vi "Check Result of the actuation.vi"(8 "error in":errorcluster, 10 "Actuator name":string, 11 "UTP IO Session in":T1) -> (0 "error out":errorcluster, 2 "Result":i16, 3 "UTP IO Session out":T1)   [LabVIEW 2023, in "Actuators.lvlib"]
doc: "Check result of the actuation"
uses:
  Actuators.lvlib
  <vilib>/Noffz/UTP IO/UTP IO Library/Typedefs/Session Handle.ctl
  <vilib>/Noffz/UTP IO/UTP IO Library/UTP IO Pool Session.lvclass
  <vilib>/Noffz/UTP IO/UTP IO Library/methods/poly/plc/Read PLC Variable (I16).vi
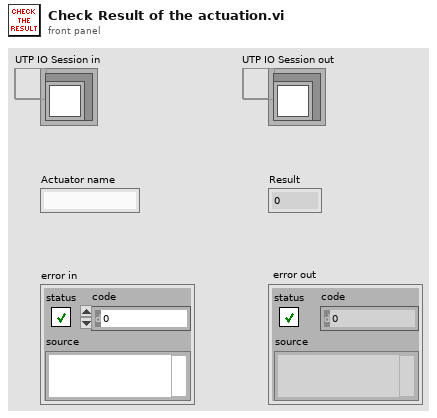
[diagram p1: front panel]
types:
  T1 = typedef "UTP IO Library.lvlib/UTP IO Pool Session.lvclass/Session Handle.ctl" = refnum<data-value>
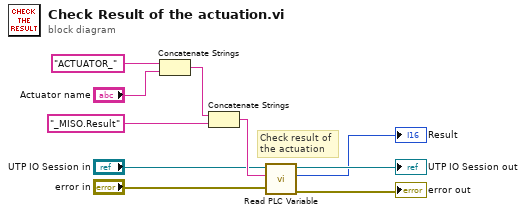
[diagram p0: block diagram]
diagram:
  # "Check result of\nthe actuation"
  n1 = Concatenate Strings("ACTUATOR_" ("string"), "Actuator name") -> (w6:string)
  n2 = Concatenate Strings(w6, "_MISO.Result" ("string")) -> (w10:string)
  n3 = call-poly <vilib>:"Read PLC Variable.vi"("error in (no error)"="error in", "variable name"=w10, "UTP IO Session in"="UTP IO Session in") -> ("error out"=→"error out":errorcluster, "value"=→"Result":i16, "UTP IO Session out"=→"UTP IO Session out":T1)  [unwired: 6 in]
